vi "AES-Mix-Columns.vi"(9 "state[i][y]":u8, 10 "state[i][x]":u8, 11 "Tmp":u8) -> (3 "state[i][x]":u8)   [LabVIEW 2017]
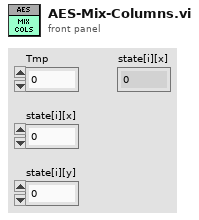
[diagram p1: front panel]
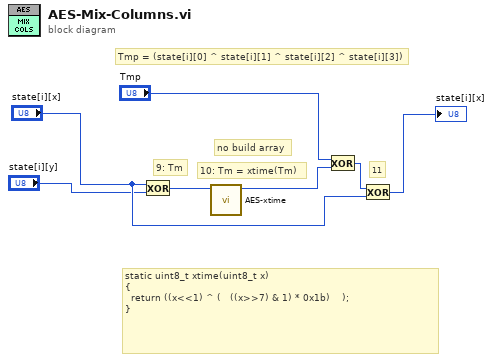
[diagram p0: block diagram]
diagram:
  # "no build array"
  # "Tmp = (state[i][0] ^ state[i][1] ^ state[i][2] ^ state[i][3])"
  # "static uint8_t xtime(uint8_t x)\n{\n  return ((x<<1) ^ (   ((x>>7) & 1) * 0x1b)    );\n}"
  # "11"
  # "10: Tm = xtime(Tm)"
  # "9: Tm"
  n1 = Exclusive Or(1:"state[i][y]", 2:"state[i][x]") -> (0:w2:u8)
  n2 = call "AES-xtime.vi"("Numeric in"=w2) -> ("Numeric out"=w4:u8)  [unwired: 10 in]
  n3 = Exclusive Or(1:w4, 2:"Tmp") -> (0:w6:u8)
  n4 = Exclusive Or(1:"state[i][x]", 2:w6) -> (0:→"state[i][x]":u8)
